vi "L0_BASELINE_TEST.vi"(7 "Serial Number":string="SN_026", 8 "error in":errorcluster, 11 "Instrument VISA in":T1={"AWG VISA"="AgilentGenerator1", "Oscilloscope  VISA "="AgilentOsciloscope", "Integration Board IP"="172.16.17.47", "connection ID"=refnum, "report out"=refnum, "report file path"=path "C:/Users/omartinez/Desktop/L0nL1_Results"}) -> (0 "error out":errorcluster, 3 "Instrument VISA out":T1={"AWG VISA"="AgilentGenerator1", "Oscilloscope  VISA "="AgilentOsciloscope", "Integration Board IP"="172.16.17.47", "connection ID"=refnum, "report out"=refnum, "report file path"=path "C:/Users/omartinez/Desktop/L0nL1_Results"})   [LabVIEW 2012]
uses:
  <vilib>/Utility/NIReport.llb/NI_report.lvclass
  <vilib>/Utility/NIReport.llb/HTML/NI_HTML.lvclass
  <instrlib>/Agilent 8000 Series/Public/Configure/Configure Math (Binary Operation).vi
  L0&L1/L0_BOARD_TESTs/trunk/Sum_Abrilader/L0_Sum_Adder Folder/C/Program Files/National Instruments/LabVIEW 2012/instr.lib/Agilent 8000 Series/Public/Data/Low Level/Fetch Measurement (More).vi
  <instrlib>/Agilent 8000 Series/Agilent 8000 Series.lvlib
panel:
  in  "finish value":i32=550
  in  "start value":i32=450
  in  "Channels":i32[](array[numeric])=[0, 1, 2, 3, 4, 5, 6]
  out "IPR_count":u32
  out "Data":string="empty_read_buffer0_2-65@1\r\n0_2-76@0\r\n"
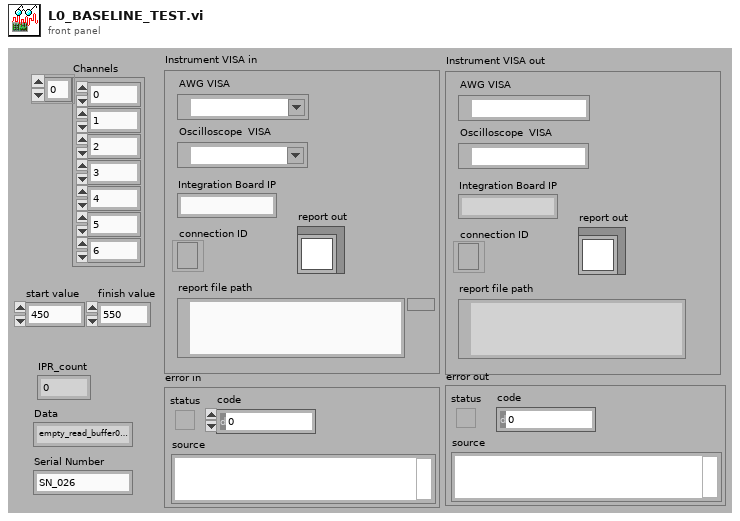
[diagram p1: front panel]
types:
  T1 = cluster{"AWG VISA":refnum<visa-resource-name>, "Oscilloscope  VISA ":refnum<visa-resource-name>, "Integration Board IP":string, "connection ID":refnum<k5>, "report out":refnum<class "NI_report.lvclass">, "report file path":path}
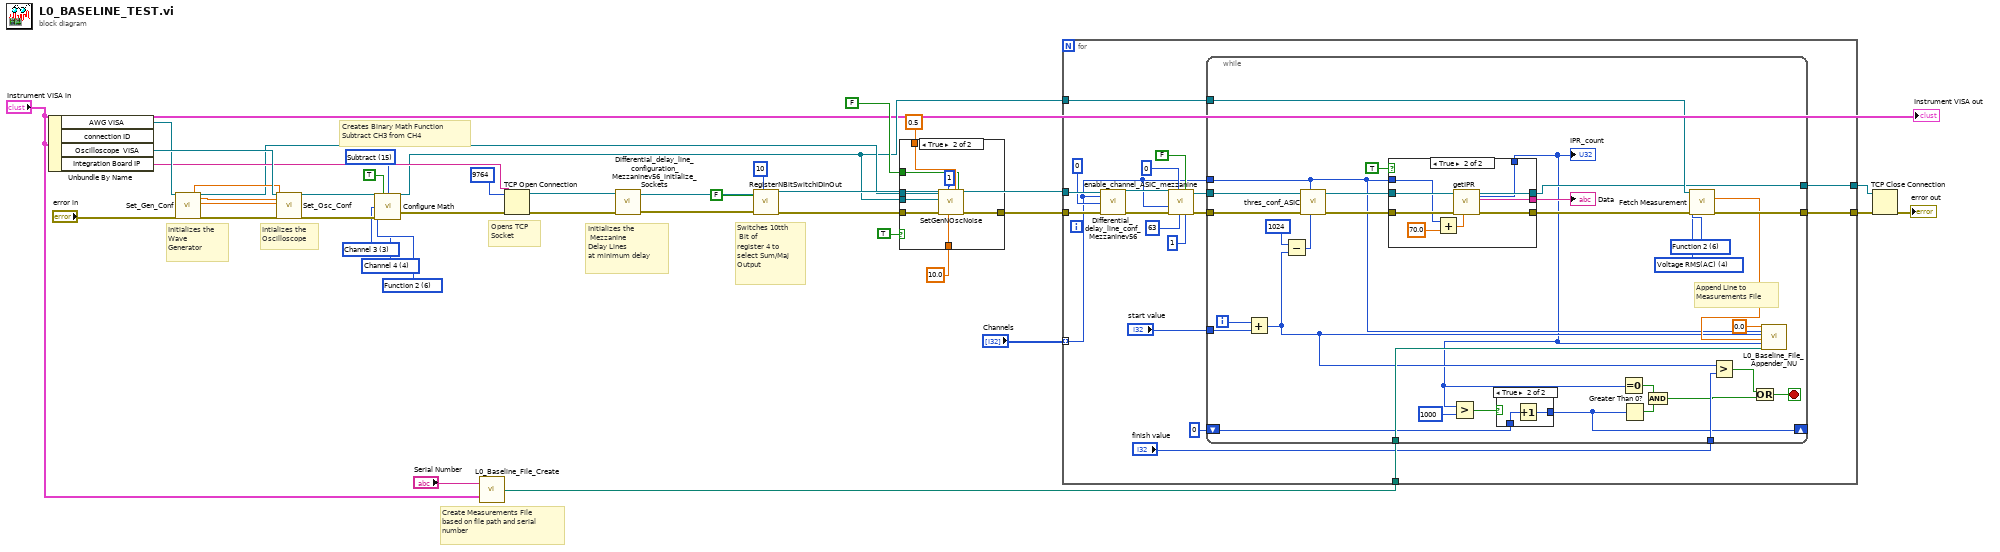
[diagram p0: block diagram]
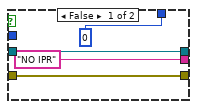
[diagram p3: hidden frame]
diagram:
  w28 = u16 6 items=["Function 1"=5, "Function 2"=6, "Function 3"=7, "Function 4"=8] ("Math Channel (5: Function 1)")
  w29 = u16 15 items=["Add"=12, "Divide"=13, "Multiply"=14, "Subtract"=15, "Common Mode"=16, "Versus"=17] ("Math Operation (12: Add)")
  w24 = 3 items=["Channel 1"=1, "Channel 2"=2, "Channel 3"=3, "Channel 4"=4] ("Channel (1: Channel 1)")
  w25 = 4 items=["Channel 1"=1, "Channel 2"=2, "Channel 3"=3, "Channel 4"=4] ("Channel (1: Channel 1)")
  # "Create Measurements File\nbased on file path and serial\nnumber"
  # "Initializes the\n Mezzanine\nDelay Lines \nat minimum delay"
  # "Switches 10tth \n Bit of\nregister 4 to \nselect Sum/Maj\nOutput"
  # "Opens TCP\nSocket"
  # "Creates Binary Math Function\nSubtract CH3 from CH4"
  # "Intializes the\nOscilloscope"
  # "Initializes the \nWave\nGenerator"
  n1 = Unbundle By Name("Instrument VISA in") -> ("AWG VISA"=w36:refnum<visa-resource-name>, "Oscilloscope  VISA"=w37:refnum<visa-resource-name>, "Integration Board IP"=w31:string)  [unwired: 1 out]
  n2 = call "Set_Gen_Conf.vi"("AWG VISA"=w36, "error in (no error)"="error in") -> ("Amplitude 1 OUT"=w34:dbl, "VISA resource name out"=w9:refnum<visa-resource-name>, "Pulse Width in seconds 1 OUT"=w33:dbl, "Trigger Level 1"=w32:dbl, "error out"=w38:errorcluster)  [unwired: 10 in, 3 out]
  n3 = call "Set_Osc_Conf.vi"("VISA resource name"=w37, "Amplitude IN"=w34, "Trigger Level IN"=w32, "Pulse Width in seconds IN"=w33, "error in (no error)"=w38) -> ("VISA resource name out"=w27:refnum<visa-resource-name>, "error out"=w26:errorcluster)  [unwired: 13 in]
  n4 = call-poly <instrlib>:"Configure Math.vi"("VISA resource name"=w27, "Enable Math Channel (T:Enable)"=TRUE, "Math Operation (12: Add)"=w29, "Math Channel (5: Function 1)"=w28, "Math Operand (1: Channel 1)"=w24, "Math Operand (2: Channel 2)"=w25, "error in (no error)"=w26) -> ("VISA resource name out"=w5:refnum<visa-resource-name>, "error out"=w19:errorcluster)  [unwired: 7 in]
  n5 = call "L0_Baseline_File_Create.vi"("input cluster"="Instrument VISA in", "Serial Number"="Serial Number") -> ("appended path"=w2:path)
  n6 = TCP Open Connection(address=w31, remote port or service name=9764, error in (no error)=w19) -> (connection ID=w16:refnum<k5>, error out=w18:errorcluster)  [unwired: 2 in]
  n7 = call "Differential_delay_line_configuration_Mezzaninev56_initialize_Sockets.vi"("connection ID"=w16, "error in (no error)"=w18) -> ("connection ID out"=w15:refnum<k5>, "error out 2"=w17:errorcluster)  [unwired: 6 in]
  n8 = call "RegisterNBitSwitchIDInOut.vi"("Switch Bit"=FALSE ("Sum/Maj 3"), "N Bit"=10, "error in (no error)"=w17, "connection ID"=w15) -> ("error out"=w22:errorcluster, "connection ID out"=w21:refnum<k5>)  [unwired: 5 in]
  n9 = case shown="True" TRUE ("Control\nGenNOsc") {
    tunnel: [w40 w48] -> w8
    tunnel: 0.5 ("Voltage Input") -> [_ w47]
    tunnel: 10.0 ("Amp Scaler 2") -> [_ w46]
    tunnel: FALSE ("Gen Active 2") -> [_ w45]
    tunnel: w5 -> [_ w44]
    tunnel: w9 -> [_ w43]
    tunnel: w22 -> [w40 w42]
    frame False {
    }
    frame True {
      n10 = call "SetGenNOscNoise.vi"("Enable Output"=w45, "Input Voltage"=w47, "Amp Scaler"=w46, "NChannels"=1, "error in (no error)"=w42, "Oscilloscope VISA"=w44, "Generator VISA"=w43) -> ("error out 2"=w48:errorcluster)  [unwired: 4 in]
    }
  }
  n11 = for {
    tunnel: w21 -> [w67]
    tunnel: w8 -> [w57]
    tunnel: [w56] -> w6
    tunnel: w5 -> [w55]
    tunnel: "Channels" -> [w54] mode=indexing
    tunnel: [w53] -> w3
    tunnel: w2 -> [w52]
    n12 = call "Differential_delay_line_conf_Mezzaninev56.vi"("connection ID"=w67, "channel"=w54, "Delay value"=0 ("Delay Enable"), "error in (no error)"=w57) -> ("connection ID out"=w65:refnum<k5>, "error out 2"=w66:errorcluster)  [unwired: 4 in, 6 out]
    n13 = call "enable_channel_ASIC_mezzanine.vi"("Clip_sel_b"=1 ("Clipping Select"), "maj/sum"=FALSE ("Sum/Maj 2"), "Ib_clipVb"=63 ("Ib Clip select"), "Att gain"=0 ("Attenuation Select"), "error in"=w66, "Channel"=w54, "connection ID"=w65) -> ("error out"=w59:errorcluster, "connection ID out"=w58:refnum<k5>)  [unwired: 2 in, 1 out]
    n14 = while {
      tunnel: w59 -> [w96]
      tunnel: w58 -> [w95]
      tunnel: [w88] -> w56
      tunnel: w55 -> [w87]
      tunnel: w54 -> [w83]
      tunnel: [w86] -> w53
      tunnel: w52 -> [w85]
      tunnel: "start value" -> [w80]
      tunnel: "finish value" -> [w79]
      shift-right: [w70] -> _
      shift-left: i16 0 ("x") -> [w71]
      i -> [w81]
      stop <- w73 stop-if-true
      w90 = 4 items=["Rise Time", "Fall Time", "Frequency", "Period", "Voltage RMS(AC)", "Voltage RMS(DC)", "Voltage RMS (AC,cycle)", "Voltage RMS (DC,cycle)", "Voltage Max", "Voltage Min", "Voltage Middle", "Voltage Vpp", "Voltage High", "Voltage Low", "Voltage Average", "Voltage Average (cycle)", "Width Negative", "Width Positive", "Duty Cycle Positive", "Amplitude", "Overshoot", "Preshoot", "Voltage Base", "Voltage Upper", "Time Max", "Time Min", "Color Grade Crossing", "Color Grade Eye Width", "Color Grade Eye Height", "Color Grade Eye Q-Factory", "Color Grade Eye Duty Cycle Distortion(Percent)", "Color Grade Eye Duty Cycle Distortion(Time)", "Color Grade Eye Jitter(PP)", "Color Grade Eye Width(RMS)", "Cycle-cycle Duty Jitter(Rising)", "Cycle-cycle Duty Jitter(Falling)", "Cycle-cycle Jitter(Rising)", "Cycle-cycle Jitter(Falling)", "Cycle-cycle - Width", "Cycle-cycle + Width", "Date Rate", "Unit Interval", "FFT Delta Frequency", "FFT Delta Magnitude", "FFT Frequency", "FFT Magnitude", "Slew Rate", "Area (Entire Display)", "Area(Single Cycle)", "Duty Cycle (Rising)", "Duty Cycle (Falling)"] ("Measurement Function (0: Rise Time)")
      w91 = 6 items=["Channel 1"=1, "Channel 2"=2, "Channel 3"=3, "Channel 4"=4, "Function 1"=5, "Function 2"=6, "Function 3"=7, "Function 4"=8, "Memory 1"=9, "Memory 2"=10, "Memory 3"=11, "Memory 4"=12] ("Channel (1: Channel 1)")
      # "Append Line to \nMeasurements File"
      n15 = Add(x=w81, y=w80) -> (x+y=w78:i32)
      n16 = Subtract(x=i16 1024, y=w78) -> (x-y=w93:i32)
      n17 = call "thres_conf_ASIC.vi"("threshold"=w93, "Ring"=w83, "error out 3"=w96, "connection ID"=w95) -> ("error out 2"=w94:errorcluster, "connection ID out"=w97:refnum<k5>)  [unwired: 4 in, 2 out]
      n18 = case shown="True" TRUE ("IPR?") {
        tunnel: w94 -> [w106 w115]
        tunnel: [w106 w107] -> w89
        tunnel: w97 -> [w105 w114]
        tunnel: [w105 w113] -> w86
        tunnel: [u32 0 ("IPR_count") w110] -> w69
        tunnel: ["NO IPR" ("Data") w109] -> w99
        tunnel: w83 -> [_ w108]
        frame False {
        }
        frame True {
          n19 = Add(x=w108, y=70.0) -> (x+y=w112:dbl)
          n20 = call "getIPR.vi"("Address"=w112, "error in"=w115, "connection ID"=w114) -> ("error out"=w107:errorcluster, "Data"=w109:string, "connection ID out"=w113:refnum<k5>, "IPR_count"=w110:u32)  [unwired: 5 in]
        }
      }
      "IPR_count" <- w69
      "Data" <- w99
      n21 = Greater?(x=w69, y=u32 1000) -> (0:w77:bool)
      n22 = case shown="True" w77 {
        tunnel: w71 -> [w100 w102]
        tunnel: [w100 w101] -> w70
        frame False {
        }
        frame True {
          n23 = Increment(x=w102) -> (x+1=w101:i16)
        }
      }
      n24 = Equal To 0?(x=w69) -> (x = 0?=w76:bool)
      n25 = Greater Than 0?(x=w70) -> (x > 0?=w75:bool)
      n26 = And(x=w76, y=w75) -> (x .and. y?=w72:bool)
      n27 = call-poly "Fetch Measurement.vi"("VISA resource name"=w87, "Channel (1: Channel 1)"=w91, "Measurement Function (0: Rise Time)"=w90, "error in (no error)"=w89) -> ("Measurement"=w84:dbl, "error out"=w88:errorcluster)  [unwired: 9 in, 1 out]
      n28 = Greater?(x=w78, y=w79) -> (0:w74:bool)
      n29 = Or(x=w74, y=w72) -> (x .or. y?=w73:bool)
      n30 = call "L0_Baseline_File_Appender_NU.vi"("Vin"=0.0, "CH"=w83, "DAC Level"=w78, "Vmeas"=w84, "IPR"=w69, "file path (dialog if empty)"=w85) -> ()  [unwired: 14 in]
    }
  }
  n31 = TCP Close Connection(connection ID=w3, error in (no error)=w6) -> (error out=→"error out":errorcluster)  [unwired: 1 in, 1 out]
  "Instrument VISA out" <- "Instrument VISA in"
